vi "Event Handler.vi"(0 "uService Template in":refnum<class "Scheduler.lvclass">=refnum, 5 "Event type":T1=enum."Message", 7 "Item Name":string, 9 "Data":variant, 11 "error in (no error)":errorcluster) -> (4 "uService Template out":refnum<class "Scheduler.lvclass">, 15 "error out":errorcluster)   [LabVIEW 2020, in "CIRCUS_uServices.lvlib" / "Scheduler.lvlib" / "Scheduler.lvclass"]
doc: "This VI is the event handler of the uService: every time an event is triggered to the uService, this VI is called.\nNote: here you can access the Actor/Class data, but it will be the one coming out from Init. You cannot modify the values.\nThree different events are supported:\nI) Button Pressed: get called on a GUI button pressed. Item Name is the name (label) of the button, Data is empty.\nII) Shared Variable Updated: get called when a SV you subscribed to is updated. Item Name is the name of the SV, and Data is the value (note: you need to convert it to the proper type).\nIII) Message: get called every time a user event is generated using Send Message to Event Handler. The values of Item Name and Data are the one given to the Send Message to Event Handler.\nIV) Ready to launch?: this frame get called every time a new Run is initiated. Each uService is responsible of performing a self check before giving back the green light for the Run to start."
uses:
  Scheduler.lvclass
  Scheduler.lvclass/Scheduler.ctl
  C:/Users/marco/Documents/GitHub_Lab/CIRCUS/TALOS/TALOS_PPL.lvlibp/Father of all uServices/Father of all uServices/Father of all uServices.lvclass
  C:/Users/marco/Documents/GitHub_Lab/CIRCUS/TALOS/TALOS_PPL.lvlibp/Ancestor/Ancestor/Ancestor.lvclass
  C:/Users/marco/Documents/GitHub_Lab/CIRCUS/TALOS/Actor Framework.lvlibp/1abvi3w/vi.lib/ActorFramework/Actor/Actor.lvclass
  C:/Users/marco/Documents/GitHub_Lab/CIRCUS/CIRCUS uServices et al/Scheduler/Scheduler.lvclass
  Scheduler Consumer Case Selector.ctl
  Add RUN Window.vi
  Scheduler.lvlib
  Preview.vi
  Get File Path for Load and Save.vi
  Run Utilities/Sequence of SBlocks/Sequence of SBlocks.lvclass
  TALOS/TALOS_PPL.lvlibp
  TALOS/TALOS_PPL.lvlibp/Father of all uServices/Father of all uServices/Father of all uServices.lvclass
  Run Utilities/Schedule/Schedule.lvclass
  TALOS/TALOS_PPL.lvlibp/Father of all uServices/Father of all uServices/Event Handler Items.ctl
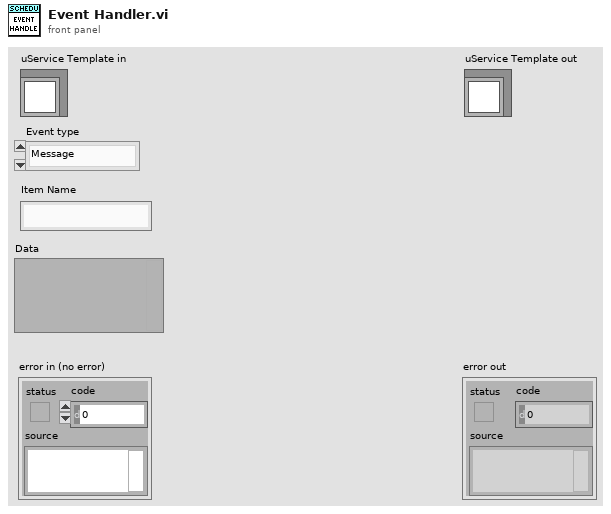
[diagram p1: front panel]
types:
  T1 = typedef "TALOS_PPL.lvlibp/Father of all uServices.lvlib/Father of all uServices.lvclass/Event Handler Items.ctl" = enum16{"Button Pressed", "Shared Variable Updated", "Message", "Ready to launch?", "Safe Mode", "Start RUN", "Stop RUN"}
  T2 = enum32{"Invalid", "Standard", "Closed", "Hidden", "Minimized", "Maximized"}
  T3 = typedef "CIRCUS_uServices.lvlib/Scheduler.lvlib/Scheduler.lvclass/Scheduler Consumer Case Selector.ctl" = enum16{"Add SBlock", "Update GUI", "Move SBlock", "Select SBlock", "Update Cont.", "Load", "Save", "Reset", "Send to Tamer", "Edit SBlock", "Duplicate SBlock", "Delete SBlock", "Update SBlock", "Init", "Split/Combine Schedules", "Reschedule", "Load Parameters"}
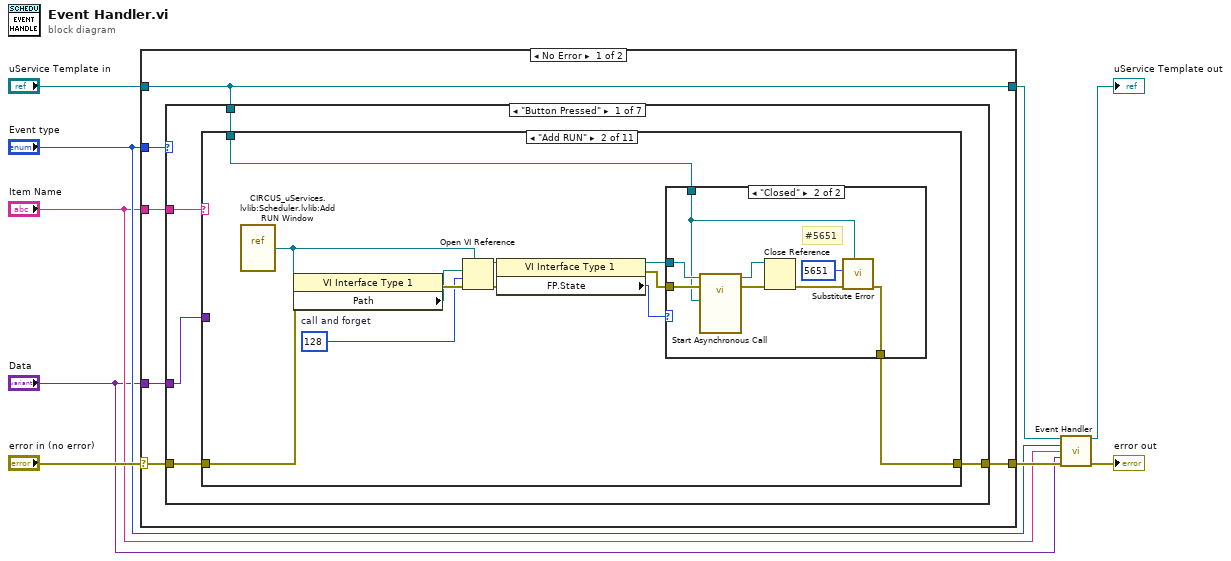
[diagram p0: block diagram]
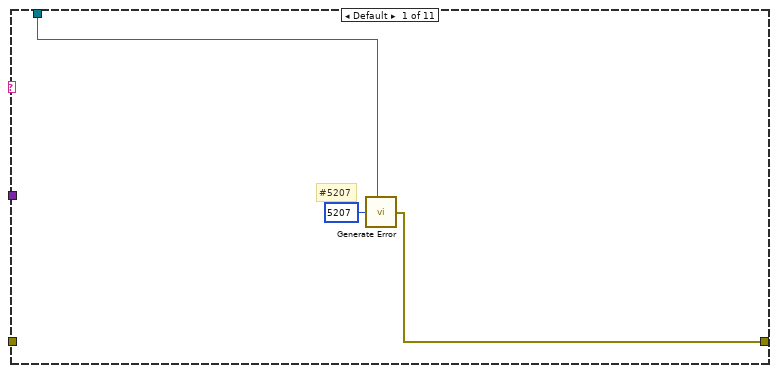
[diagram p2: hidden frame]
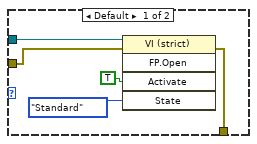
[diagram p3: hidden frame]
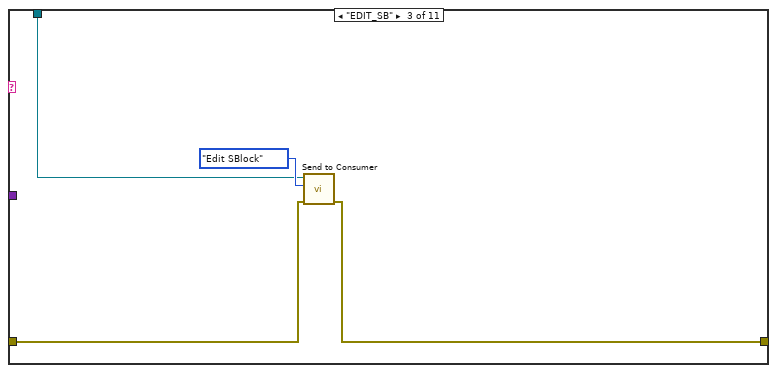
[diagram p4: hidden frame]
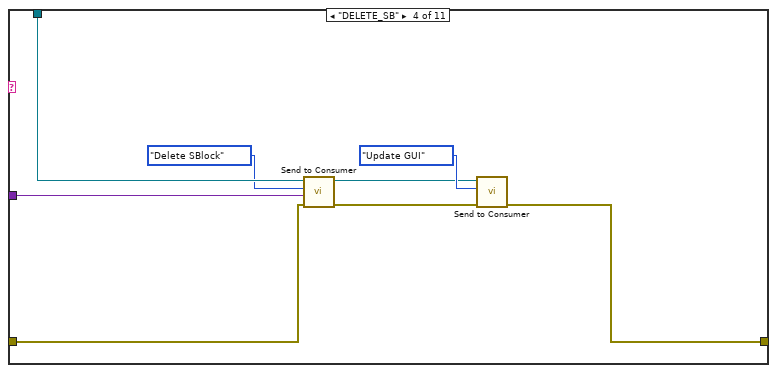
[diagram p5: hidden frame]
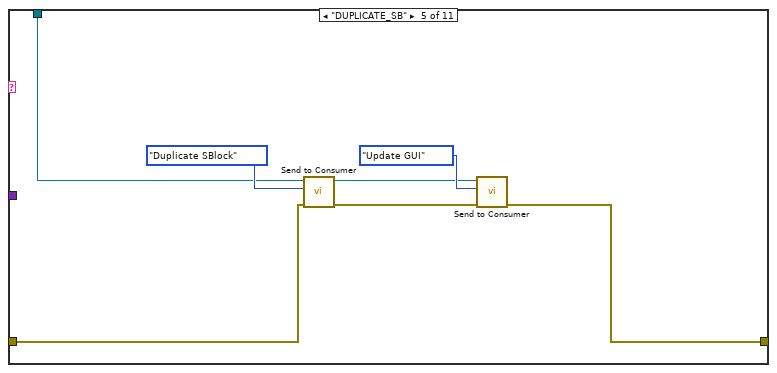
[diagram p6: hidden frame]
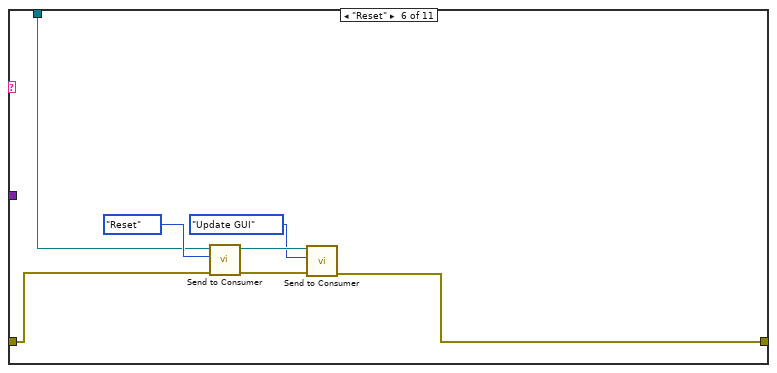
[diagram p7: hidden frame]
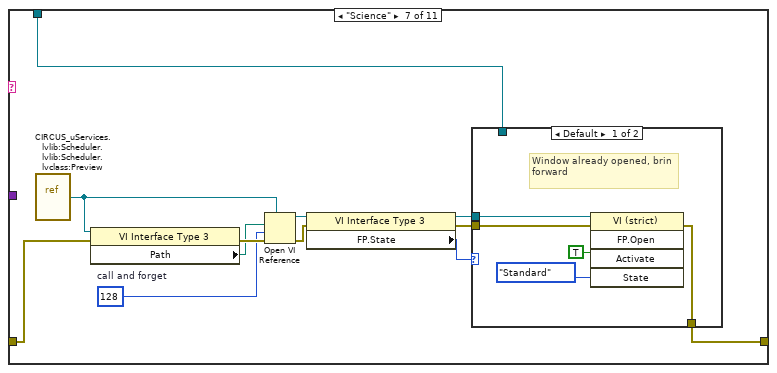
[diagram p8: hidden frame]
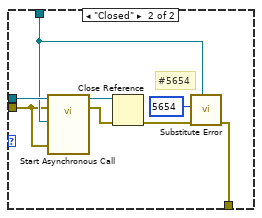
[diagram p9: hidden frame]
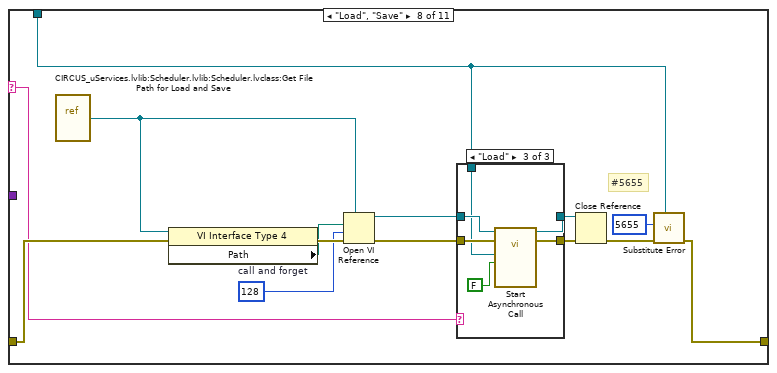
[diagram p10: hidden frame]
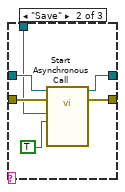
[diagram p12: hidden frame]
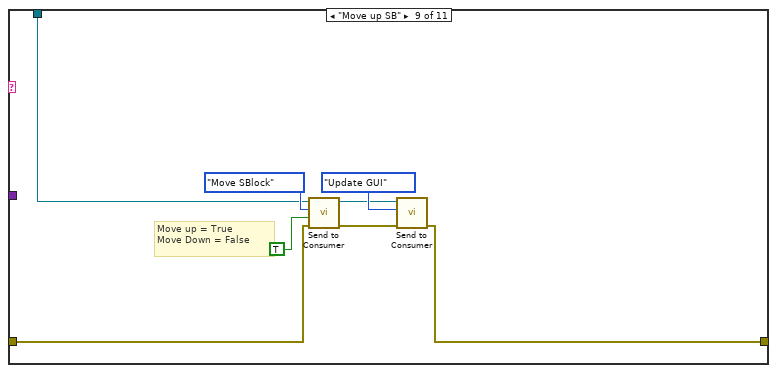
[diagram p13: hidden frame]
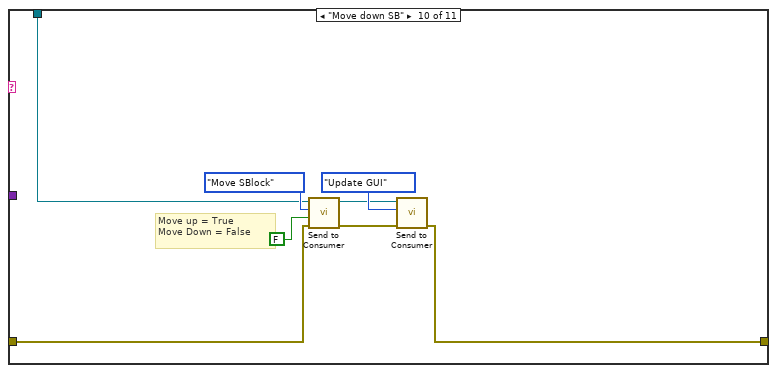
[diagram p14: hidden frame]
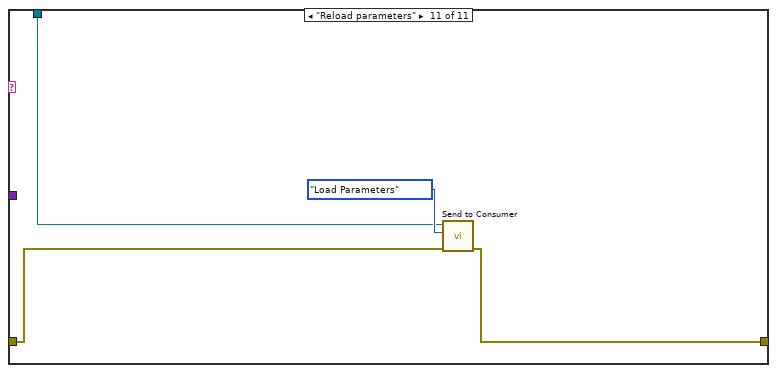
[diagram p15: hidden frame]
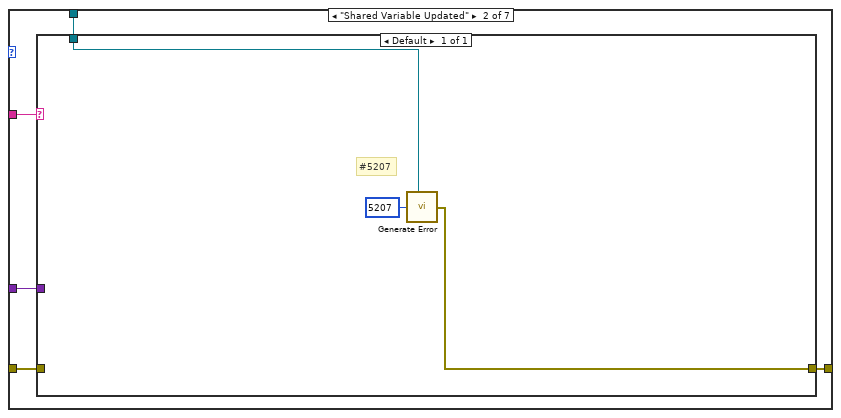
[diagram p16: hidden frame]
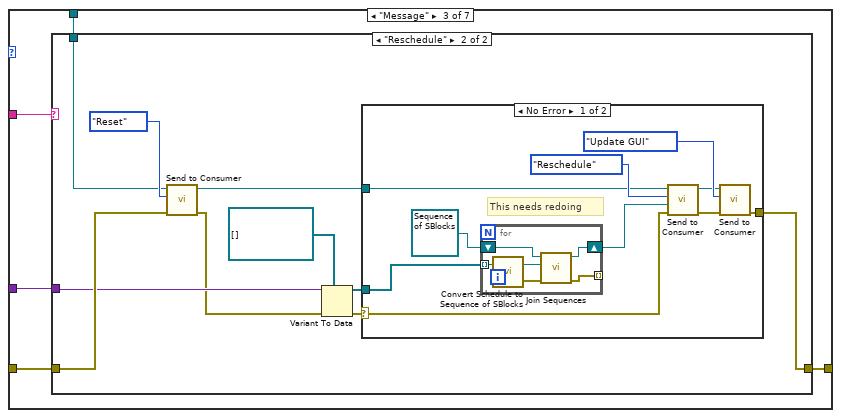
[diagram p17: hidden frame]
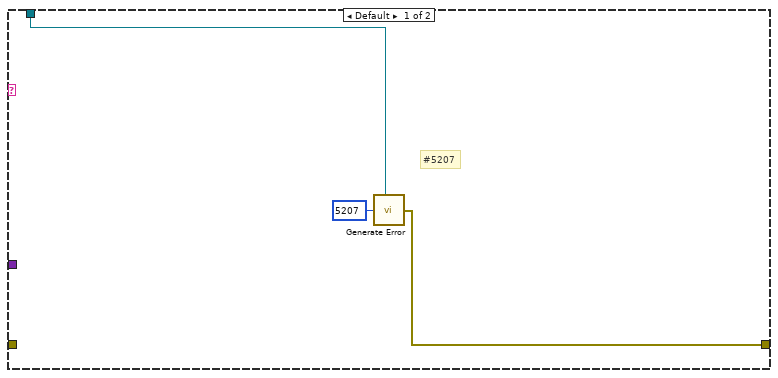
[diagram p18: hidden frame]
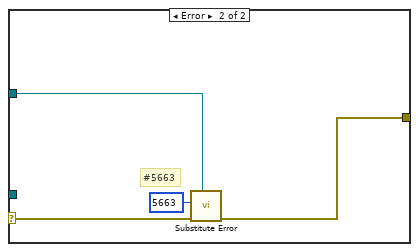
[diagram p19: hidden frame]
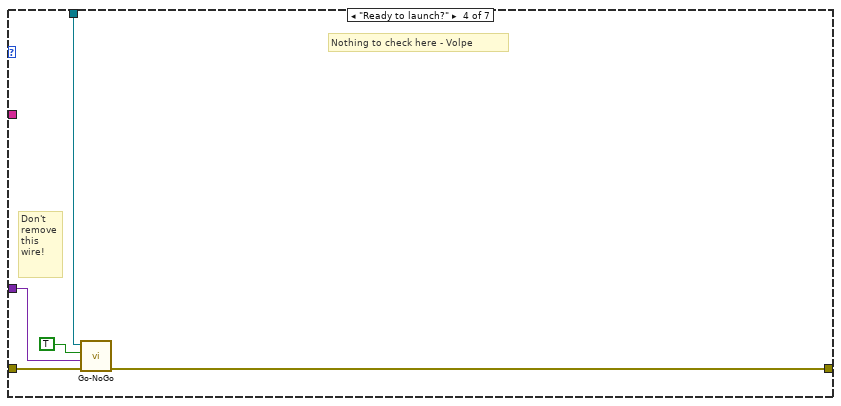
[diagram p20: hidden frame]
diagram:
  n1 = case shown="No Error" "error in (no error)" {
    selector: "error in (no error)" -> [w13 w203]
    tunnel: [w14 w203] -> w7
    tunnel: [w12 w202] -> w4
    tunnel: "uService Template in" -> [w12 w202]
    tunnel: "Event type" -> [w15 _]
    tunnel: "Item Name" -> [w11 _]
    tunnel: "Data" -> [w10 _]
    frame No Error {
      n2 = case shown="\"Button Pressed\"" w15 {
        tunnel: [w20 w148 w156 w197 w199 w200 w201] -> w14
        tunnel: w13 -> [w17 w150 w160 w198 w199 w200 w201]
        tunnel: w11 -> [w18 w152 w159 _ _ _ _]
        tunnel: w12 -> [w19 w149 w157 w196 _ _ _]
        tunnel: w10 -> [w16 w151 w158 w194 _ _ _]
        frame "Button Pressed" {
          n3 = case shown="\"Add RUN\"" w18 {
            selector: w18 -> [_ _ _ _ _ _ _ w101 _ _ _]
            tunnel: w17 -> [_ w28 w52 w60 w67 w73 w82 w105 w133 w141 w147]
            tunnel: [w21 w31 w51 w54 w63 w70 w79 w102 w132 w140 w146] -> w20
            tunnel: w19 -> [w22 w32 w49 w59 w62 w69 w81 w104 w130 w138 w144]
            tunnel: w16 -> [_ _ _ w58 _ _ _ _ _ _ _]
            frame Default {
              # "#5207"
              n4 = call "Generate Error.vi"("Class"=w22, "Error Code"=5207) -> ("error out"=w21:errorcluster)  [unwired: 5 in]
            }
            frame "Add RUN" {
              w33 = 128  # call and forget
              n5 = vi-ref "CIRCUS_uServices.lvlib:Scheduler.lvlib:Add RUN Window.vi"() -> (w30:refnum<vi>)
              n6 = property class="VI Interface Type 1"(reference=w30, error in=w28) -> (error out=w35:errorcluster, "Path"=w29:path)  [unwired: 1 out]
              n7 = Open VI Reference(type specifier VI Refnum (for type only)=w30, vi path=w29, options=w33, error in (no error)=w35) -> (vi reference=w34:refnum<vi>, error out=w26:errorcluster)  [unwired: 2 in]
              n8 = property class="VI Interface Type 1"(reference=w34, error in=w26) -> (reference out=w27:refnum<vi>, error out=w25:errorcluster, "FP.State"=w24:T2)
              n9 = case shown="\"Closed\"" w24 {
                tunnel: w25 -> [w39 w48]
                tunnel: w27 -> [w40 w46]
                tunnel: w32 -> [_ w41]
                tunnel: [w38 w43] -> w31
                frame Default {
                  n10 = invoke class="VI (strict)" method="FP.Open"(reference=w40, error in=w39, "Activate"=TRUE ("Activate?"), "State"=T2."Standard") -> (error out=w38:errorcluster)  [unwired: 1 in, 4 out]
                }
                frame "Closed" {
                  # "#5651"
                  n11 = call-by-ref "Start Asynchronous Call"(reference=w46, error in=w48, "Scheduler in"=w41) -> (reference out=w45:refnum<vi>, error out=w47:errorcluster)  [unwired: 9 in, 2 out]
                  n12 = Close Reference(reference=w45, error in (no error)=w47) -> (error out=w44:errorcluster)
                  n13 = call "Substitute Error.vi"("LabVIEW Object"=w41, "error in (no error)"=w44, "Error Code"=5651) -> ("error out"=w43:errorcluster)  [unwired: 8 in]
                }
              }
            }
            frame "EDIT_SB" {
              n14 = call "Send to Consumer.vi"("error in (no error)"=w52, "Case ID"=Scheduler_Consumer_Case_Selector."Edit SBlock" ("Shifter Panel Consumer Case Selector"), "uService Template in"=w49) -> ("error out"=w51:errorcluster)  [unwired: 7 in, 1 out]
            }
            frame "DELETE_SB" {
              n15 = call "Send to Consumer.vi"("error in (no error)"=w60, "Data"=w58, "Case ID"=Scheduler_Consumer_Case_Selector."Delete SBlock" ("Shifter Panel Consumer Case Selector"), "uService Template in"=w59) -> ("error out"=w55:errorcluster, "uService Template out"=w53:refnum<class "Scheduler.lvclass">)  [unwired: 6 in]
              n16 = call "Send to Consumer.vi"("error in (no error)"=w55, "Case ID"=Scheduler_Consumer_Case_Selector."Update GUI" ("Shifter Panel Consumer Case Selector"), "uService Template in"=w53) -> ("error out"=w54:errorcluster)  [unwired: 7 in, 1 out]
            }
            frame "DUPLICATE_SB" {
              n17 = call "Send to Consumer.vi"("error in (no error)"=w67, "Case ID"=Scheduler_Consumer_Case_Selector."Duplicate SBlock" ("Shifter Panel Consumer Case Selector"), "uService Template in"=w62) -> ("error out"=w64:errorcluster, "uService Template out"=w61:refnum<class "Scheduler.lvclass">)  [unwired: 7 in]
              n18 = call "Send to Consumer.vi"("error in (no error)"=w64, "Case ID"=Scheduler_Consumer_Case_Selector."Update GUI" ("Shifter Panel Consumer Case Selector"), "uService Template in"=w61) -> ("error out"=w63:errorcluster)  [unwired: 7 in, 1 out]
            }
            frame "Reset" {
              n19 = call "Send to Consumer.vi"("error in (no error)"=w73, "Case ID"=Scheduler_Consumer_Case_Selector."Reset" ("Shifter Panel Consumer Case Selector"), "uService Template in"=w69) -> ("error out"=w71:errorcluster, "uService Template out"=w72:refnum<class "Scheduler.lvclass">)  [unwired: 7 in]
              n20 = call "Send to Consumer.vi"("error in (no error)"=w71, "Case ID"=Scheduler_Consumer_Case_Selector."Update GUI" ("Shifter Panel Consumer Case Selector"), "uService Template in"=w72) -> ("error out"=w70:errorcluster)  [unwired: 7 in, 1 out]
            }
            frame "Science" {
              w83 = 128  # call and forget
              n21 = vi-ref "CIRCUS_uServices.lvlib:Scheduler.lvlib:Scheduler.lvclass:Preview.vi"() -> (w80:refnum<vi>)
              n22 = property class="VI Interface Type 3"(reference=w80, error in=w82) -> (error out=w86:errorcluster, "Path"=w85:path)  [unwired: 1 out]
              n23 = Open VI Reference(type specifier VI Refnum (for type only)=w80, vi path=w85, options=w83, error in (no error)=w86) -> (vi reference=w84:refnum<vi>, error out=w77:errorcluster)  [unwired: 2 in]
              n24 = property class="VI Interface Type 3"(reference=w84, error in=w77) -> (reference out=w78:refnum<vi>, error out=w76:errorcluster, "FP.State"=w75:T2)
              n25 = case shown="Default" w75 {
                tunnel: w81 -> [_ w93]
                tunnel: [w87 w96] -> w79
                tunnel: w78 -> [w89 w94]
                tunnel: w76 -> [w88 w92]
                frame Default {
                  # "Window already opened, brin forward"
                  n26 = invoke class="VI (strict)" method="FP.Open"(reference=w89, error in=w88, "Activate"=TRUE ("Activate?"), "State"=T2."Standard") -> (error out=w87:errorcluster)  [unwired: 1 in, 4 out]
                }
                frame "Closed" {
                  # "#5654"
                  n27 = call-by-ref "Start Asynchronous Call"(reference=w94, error in=w92, 8:"error in (no error)"=w92, "Scheduler in"=w93) -> (reference out=w98:refnum<vi>, error out=w97:errorcluster)  [unwired: 8 in, 2 out]
                  n28 = Close Reference(reference=w98, error in (no error)=w97) -> (error out=w99:errorcluster)
                  n29 = call "Substitute Error.vi"("LabVIEW Object"=w93, "error in (no error)"=w99, "Error Code"=5654) -> ("error out"=w96:errorcluster)  [unwired: 8 in]
                }
              }
            }
            frame "Load", "Save" {
              w106 = 128  # call and forget
              # "#5655"
              n30 = vi-ref "CIRCUS_uServices.lvlib:Scheduler.lvlib:Scheduler.lvclass:Get File Path for Load and Save.vi"() -> (w103:refnum<vi>)
              n31 = property class="VI Interface Type 4"(reference=w103, error in=w105) -> (error out=w113:errorcluster, "Path"=w112:path)  [unwired: 1 out]
              n32 = Open VI Reference(type specifier VI Refnum (for type only)=w103, vi path=w112, options=w106, error in (no error)=w113) -> (vi reference=w109:refnum<vi>, error out=w107:errorcluster)  [unwired: 2 in]
              n33 = case shown="\"Load\"" w101 {
                tunnel: [w115 w116 w127] -> w110
                tunnel: w109 -> [w115 w121 w126]
                tunnel: [w114 w120 w125] -> w108
                tunnel: w107 -> [w114 w119 w124]
                tunnel: w104 -> [_ w118 w123]
                frame Default {
                }
                frame "Save" {
                  n34 = call-by-ref "Start Asynchronous Call"(reference=w121, error in=w119, "Save/Load"=TRUE, "Scheduler in"=w118) -> (reference out=w116:refnum<vi>, error out=w120:errorcluster)  [unwired: 8 in, 2 out]
                }
                frame "Load" {
                  n35 = call-by-ref "Start Asynchronous Call"(reference=w126, error in=w124, "Save/Load"=FALSE, "Scheduler in"=w123) -> (reference out=w127:refnum<vi>, error out=w125:errorcluster)  [unwired: 8 in, 2 out]
                }
              }
              n36 = Close Reference(reference=w110, error in (no error)=w108) -> (error out=w111:errorcluster)
              n37 = call "Substitute Error.vi"("LabVIEW Object"=w104, "error in (no error)"=w111, "Error Code"=5655) -> ("error out"=w102:errorcluster)  [unwired: 8 in]
            }
            frame "Move up SB" {
              # "Move up = True\nMove Down = False"
              n38 = call "Send to Consumer.vi"("error in (no error)"=w133, "Data"=TRUE, "Case ID"=Scheduler_Consumer_Case_Selector."Move SBlock" ("Shifter Panel Consumer Case Selector"), "uService Template in"=w130) -> ("error out"=w131:errorcluster, "uService Template out"=w129:refnum<class "Scheduler.lvclass">)  [unwired: 6 in]
              n39 = call "Send to Consumer.vi"("error in (no error)"=w131, "Case ID"=Scheduler_Consumer_Case_Selector."Update GUI" ("Shifter Panel Consumer Case Selector"), "uService Template in"=w129) -> ("error out"=w132:errorcluster)  [unwired: 7 in, 1 out]
            }
            frame "Move down SB" {
              # "Move up = True\nMove Down = False"
              n40 = call "Send to Consumer.vi"("error in (no error)"=w141, "Data"=FALSE, "Case ID"=Scheduler_Consumer_Case_Selector."Move SBlock" ("Shifter Panel Consumer Case Selector"), "uService Template in"=w138) -> ("error out"=w139:errorcluster, "uService Template out"=w137:refnum<class "Scheduler.lvclass">)  [unwired: 6 in]
              n41 = call "Send to Consumer.vi"("error in (no error)"=w139, "Case ID"=Scheduler_Consumer_Case_Selector."Update GUI" ("Shifter Panel Consumer Case Selector"), "uService Template in"=w137) -> ("error out"=w140:errorcluster)  [unwired: 7 in, 1 out]
            }
            frame "Reload parameters" {
              n42 = call "Send to Consumer.vi"("error in (no error)"=w147, "Case ID"=Scheduler_Consumer_Case_Selector."Load Parameters" ("Shifter Panel Consumer Case Selector"), "uService Template in"=w144) -> ("error out"=w146:errorcluster)  [unwired: 7 in, 1 out]
            }
          }
        }
        frame "Shared Variable Updated" {
          n43 = case shown="Default" w152 {
            tunnel: w151 -> [_]
            tunnel: w150 -> [_]
            tunnel: w149 -> [w154]
            tunnel: [w153] -> w148
            frame Default {
              # "#5207"
              n44 = call "Generate Error.vi"("Class"=w154, "Error Code"=5207) -> ("error out"=w153:errorcluster)  [unwired: 5 in]
            }
          }
        }
        frame "Message" {
          n45 = case shown="\"Reschedule\"" w159 {
            tunnel: w160 -> [_ w172]
            tunnel: w158 -> [_ w171]
            tunnel: w157 -> [w162 w164]
            tunnel: [w161 w173] -> w156
            frame Default {
              # "#5207"
              n46 = call "Generate Error.vi"("Class"=w162, "Error Code"=5207) -> ("error out"=w161:errorcluster)  [unwired: 5 in]
            }
            frame "Reschedule" {
              n47 = call "Send to Consumer.vi"("error in (no error)"=w172, "Case ID"=Scheduler_Consumer_Case_Selector."Reset" ("Shifter Panel Consumer Case Selector"), "uService Template in"=w164) -> ("error out"=w168:errorcluster, "uService Template out"=w170:refnum<class "Scheduler.lvclass">)  [unwired: 7 in]
              n48 = Variant To Data(error in=w168, type=refnum<class "Schedule.lvclass">[] [], Variant=w171) -> (data=w166:refnum<class "Schedule.lvclass">[], error out=w165:errorcluster)
              n49 = case shown="No Error" w165 {
                selector: w165 -> [w178 w191]
                tunnel: [w176 w192] -> w173
                tunnel: w170 -> [w182 w193]
                tunnel: w166 -> [w181 _]
                frame No Error {
                  # "This needs redoing"
                  n50 = for {
                    tunnel: w181 -> [w189] mode=indexing
                    shift-right: [w186] -> w179
                    shift-left: refnum<class "Sequence of SBlocks.lvclass"> refnum ("Sequence of SBlocks in") -> [w187]
                    tunnel: [w184] -> _ mode=indexing
                    n51 = call "Convert Schedule to Sequence of SBlocks.vi"("Schedule"=w189) -> ("error out"=w185:errorcluster, "Sequence of SBlocks"=w188:refnum<class "Sequence of SBlocks.lvclass">)  [unwired: 1 in]
                    n52 = call-dynamic "Join Sequences.vi"("error in (no error)"=w185, "Sequence of SBlocks"=w188, "Sequence of SBlocks in"=w187) -> ("error out"=w184:errorcluster, "Sequence of SBlocks out"=w186:refnum<class "Sequence of SBlocks.lvclass">)  [unwired: 7 in]
                  }
                  n53 = call "Send to Consumer.vi"("error in (no error)"=w178, "Data"=w179, "Case ID"=Scheduler_Consumer_Case_Selector."Reschedule" ("Shifter Panel Consumer Case Selector"), "uService Template in"=w182) -> ("error out"=w177:errorcluster, "uService Template out"=w174:refnum<class "Scheduler.lvclass">)  [unwired: 6 in]
                  n54 = call "Send to Consumer.vi"("error in (no error)"=w177, "Case ID"=Scheduler_Consumer_Case_Selector."Update GUI" ("Shifter Panel Consumer Case Selector"), "uService Template in"=w174) -> ("error out"=w176:errorcluster)  [unwired: 7 in, 1 out]
                }
                frame Error {
                  # "#5663"
                  n55 = call "Substitute Error.vi"("LabVIEW Object"=w193, "error in (no error)"=w191, "Error Code"=5663) -> ("error out"=w192:errorcluster)  [unwired: 8 in]
                }
              }
            }
          }
        }
        frame "Ready to launch?" {
          # "Nothing to check here - Volpe"
          # "Don't remove this wire!"
          n56 = call-dynamic "Go-NoGo.vi"("error in (no error)"=w198, "Go-NoGo Data"=w194, "Go?"=TRUE, "Father of all uServices in"=w196) -> ("error out"=w197:errorcluster)  [unwired: 6 in, 1 out]
        }
        frame "Safe Mode" {
          # "Do nothing - Volpe"
        }
        frame "Start RUN" {
        }
        frame "Stop RUN" {
        }
      }
    }
    frame Error {
    }
  }
  n57 = call-parent "Event Handler.vi"("uService Template in"=w4, "Event type"="Event type", "Item Name"="Item Name", "Data"="Data", "error in (no error)"=w7) -> ("uService Template out"=→"uService Template out":refnum<class "Scheduler.lvclass">, "error out"=→"error out":errorcluster)  [unwired: 9 in]
